vi "FPGA_VI.vi"() -> ()   [LabVIEW 2014]
uses:
  FPGA_Controls/AquisitionState.ctl
  <vilib>/Platform/TimedLoop/XDataNode/timing_clust.ctl
  <vilib>/Platform/TimedLoop/XDataNode/nitl_modes.ctl
  <vilib>/Platform/TimedLoop/XDataNode/wakeup.ctl
  <vilib>/rvi/Emulation/niFpgaSctlEmulationGetInTimedLoop.vi
  <vilib>/rvi/Emulation/niFpgaEmulationReportErrorSimple.vi
  <vilib>/rvi/Emulation/niFpgaGetClockAttributes.vi
  <vilib>/rvi/Emulation/niFpgaCriticalErrorInLSC.vi
  <vilib>/rvi/eio/common/nirviEmuTemplateMethod_errors.vi
  <vilib>/rvi/Emulation/niFpgaProcessEmulError.vi
  <vilib>/rvi/interface/RandomDataEmulation/niFpgaRandomDataHandleErrors.vi
  <vilib>/Platform/TimedLoop/XDataNode/XDataNode.xnode
  <vilib>/eio/EIONode/EIONode.xnode
  <vilib>/rvi/DataTransferAndStorage/Container/XNode/niFpgaContainer.xnode
  <vilib>/rvi/interface/RandomDataEmulation/nirviRandomDataFpgaReadWriteTemplate.vi
  <vilib>/Platform/TimedLoop/XDataNode/XDNodeRunTimeDep.lvlib
panel:
  in  "Trigger":bool
  out "Init Done":bool
  out "Acquisition \nState":T1=enum."Idle (Wait for Trigger)"
  # "ADC"
  # "Status"
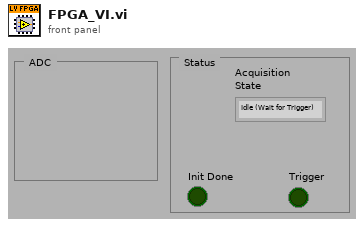
[diagram p1: front panel]
types:
  T1 = typedef "AquisitionState.ctl" = enum16{"Clear DRAM", "Idle (Wait for Trigger)", "Aquire", "Transfer DRAM Block 0", "Transfer DRAM Block 1"}
  T2 = typedef "XDNodeRunTimeDep.lvlib/timing_clust.ctl" = cluster{"Expected End [f-1]":u64, "Actual End [f-1]":u64, "Finished Late? [f-1]":bool, "Expected End [i-1]":u64, "Actual End [i-1]":u64, "Finished Late? [i-1]":bool, "Expected Start [i]":u64, "Actual Start [i]":u64, "Expected Start [f]":u64, "Actual Start [f]":u64, "Source Name":string, "Structure Name":string, "Period":i64, "Deadline":i64, "Offset":i64, "Start":i64, "Priority":i32, "Timeout":i32, "Mode":T3, "Wakeup Reason":T4, "Error":errorcluster, "Source Type":string, "Secondary Source Type":string, "Global End Time":u64, "Global Start Time":u64, "Frame Duration":u64, "Iteration Duration":u64, "Assigned CPU":i32, "I/O Scan Engine Mode":u32}
  T3 = typedef "XDNodeRunTimeDep.lvlib/nitl_modes.ctl" = enum32{"No Change", "Process missed periods, maintain original phase", "Discard missed periods, maintain original phase", "Process missed periods, ignore original phase", "Discard missed periods, ignore original phase"}
  T4 = typedef "XDNodeRunTimeDep.lvlib/wakeup.ctl" = enum32{"Normal", "Aborted", "Asynchronous wakeup", "Timing source error", "Timed loop error", "Timeout"}
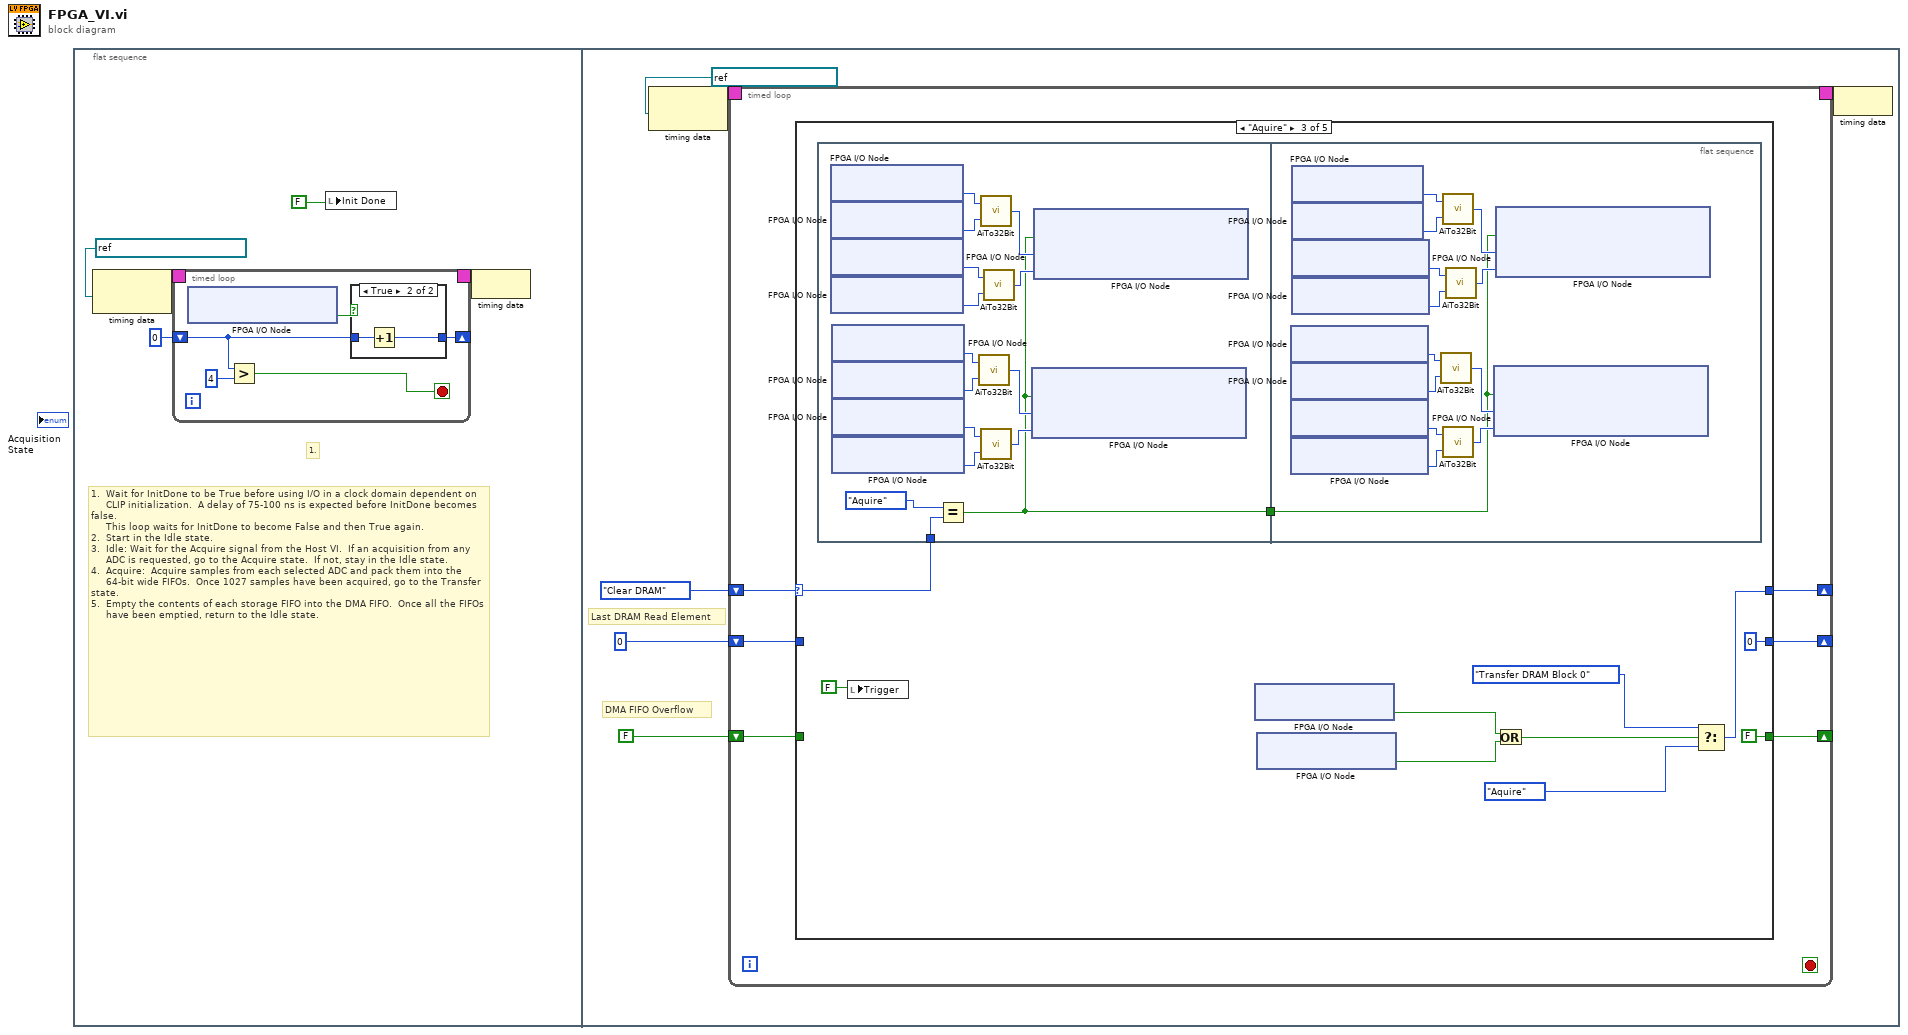
[diagram p0: block diagram]
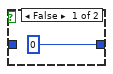
[diagram p2: hidden frame]
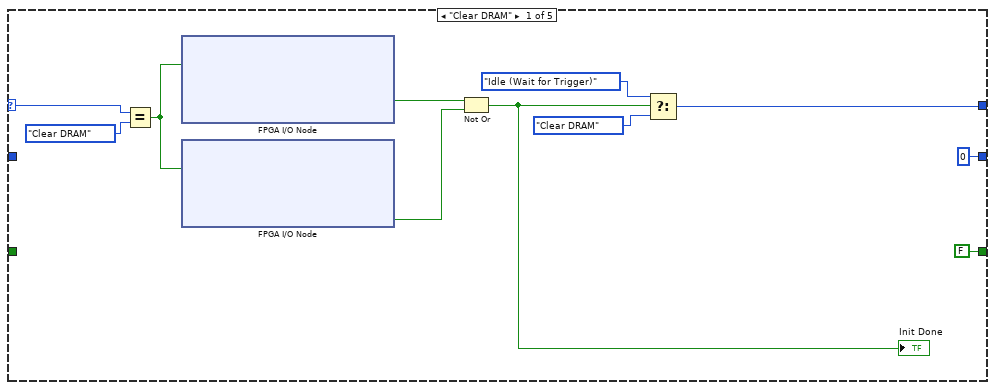
[diagram p3: hidden frame]
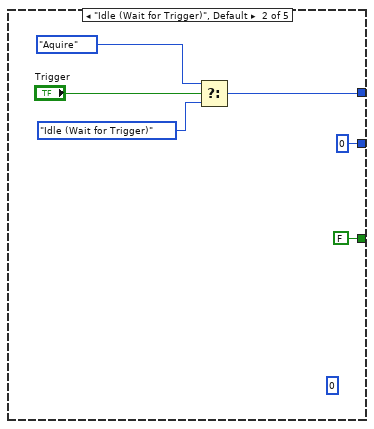
[diagram p4: hidden frame]
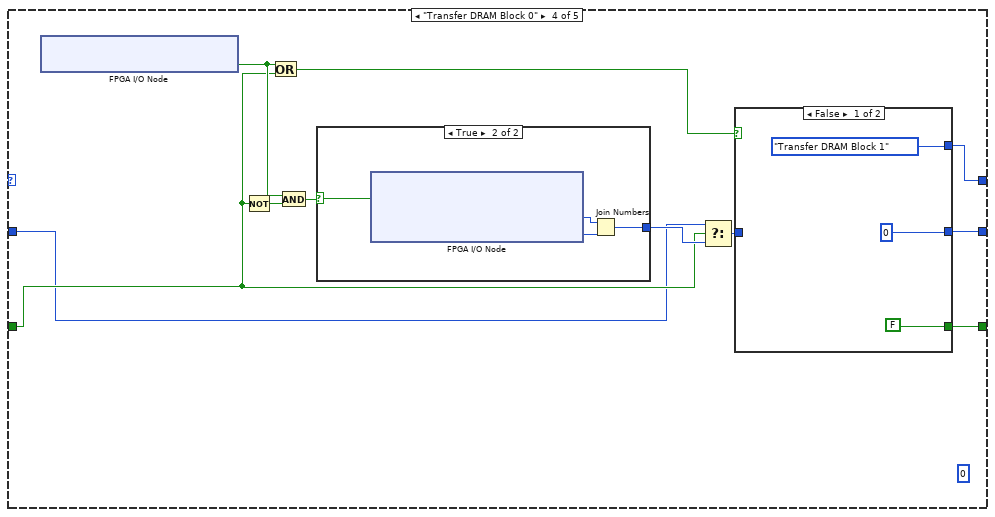
[diagram p5: hidden frame]
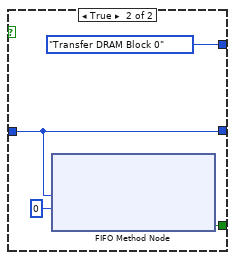
[diagram p6: hidden frame]
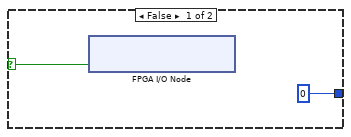
[diagram p7: hidden frame]
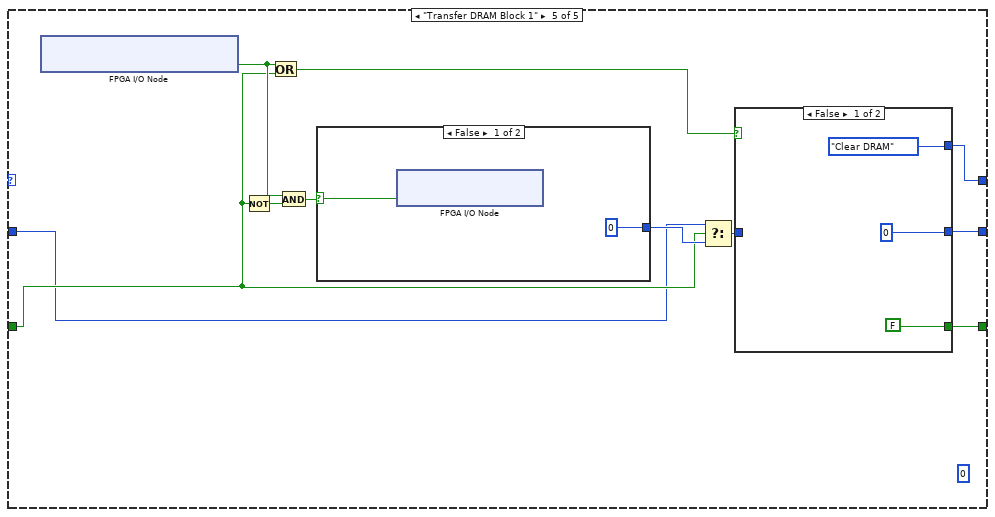
[diagram p8: hidden frame]
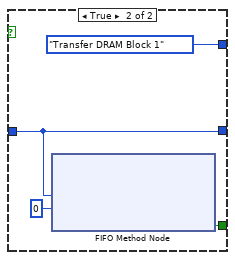
[diagram p9: hidden frame]
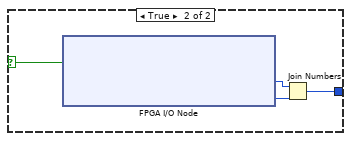
[diagram p10: hidden frame]
diagram:
  n1 = flat-sequence {
    frame #0 {
      # "1.  Wait for InitDone to be True before using I/O in a clock domain dependent on \n     CLIP initialization.  A delay of 75-100 ns is expected before InitDone becomes false.  \n     This loop waits for InitDone to become False and then True again.\n2.  Start in the Idle state. \n3.  Idle: Wait for the Acquire signal from the Host VI.  If an acquisition from any \n     ADC is requested, go to the Acquire state.  If not, stay in the Idle state.\n4.  Acquire:  Acquire samples from each selected ADC and pack them into the  \n     64-bit wide FIFOs.  Once 1027 samples have been acquired, go to the Transfer state.\n5.  Empty the contents of each storage FIFO into the DMA FIFO.  Once all the FIFOs \n     have been emptied, return to the Idle state."
      # "1."
      n2 = node-c288(refnum<k21> "40 MHz Onboard Clock" ("Source Name")) -> (w5:T2)
      n3 = timed-loop {
        shift-right: [w9] -> _
        shift-left: u16 0 -> [w8]
        timing: w5 -> [_]
        timing-out: [_] -> w4
        stop <- w6 stop-if-true
        n4 = xnode "FPGA I/O Node"() -> ("IO Module\\InitDone"=w10:bool)  [unwired: 1 in, 1 out]
        n5 = Greater?(x=w8, y=u16 4) -> (0:w6:bool)
        n6 = case shown="True" w10 {
          tunnel: [u16 0 w13] -> w9
          tunnel: w8 -> [_ w12]
          frame False {
          }
          frame True {
            n7 = Increment(x=w12) -> (x+1=w13:u16)
          }
        }
      }
      n8 = local write "Init Done"(FALSE) -> ()
      n9 = node-c288(w4) -> ()
    }
    frame #1 {
      # "Last DRAM Read Element"
      # "DMA FIFO Overflow"
      n10 = node-c288(refnum<k21> "IO Module Clock 0" ("Source Name")) -> (w25:T2)
      n11 = timed-loop {
        timing: w25 -> [_]
        timing-out: [_] -> w24
        shift-right: [w30] -> _
        shift-left: AquisitionState."Clear DRAM" ("AquistionState") -> [w31]
        shift-right: [w29] -> _
        shift-left: FALSE ("Timed Out?") -> [w27]
        shift-right: [w28] -> _
        shift-left: u64 0 ("Timeout") -> [w26]
        stop <- _ stop-if-true
        n12 = case shown="\"Aquire\"" w31 {
          selector: w31 -> [w42 _ w59 _ _]
          tunnel: [w37 w46 w55 w92 w116] -> w30
          tunnel: [FALSE ("Timed Out?") FALSE ("Timed Out?") FALSE ("Timed Out?") w93 w117] -> w29
          tunnel: [u64 0 ("Timeout") u64 0 ("Timeout") u64 0 ("Timeout") w90 w114] -> w28
          tunnel: w27 -> [_ _ _ w89 w113]
          tunnel: w26 -> [_ _ _ w88 w112]
          frame "Clear DRAM" {
            n13 = Equal?(x=w42, y=AquisitionState."Clear DRAM" ("AquistionState")) -> (x = y?=w40:bool)
            n14 = xnode "FPGA I/O Node"("DRAM Bank 0\\Read"=w40) -> ("DRAM Bank 0\\Data_Available"=w39:bool)  [unwired: 4 in, 6 out]
            n15 = xnode "FPGA I/O Node"("DRAM Bank 1\\Read"=w40) -> ("DRAM Bank 1\\Data_Available"=w38:bool)  [unwired: 4 in, 6 out]
            n16 = Not Or(1:w38, 2:w39) -> (0:w32:bool)
            "Init Done" <- w32
            n17 = Select(t=AquisitionState."Idle (Wait for Trigger)" ("AquistionState"), s=w32, f=AquisitionState."Clear DRAM" ("AquistionState")) -> (s? t:f=w37:T1)
          }
          frame "Idle (Wait for Trigger)", Default {
            (unwired) 0
            n18 = Select(t=AquisitionState."Aquire" ("AquistionState"), s="Trigger", f=AquisitionState."Idle (Wait for Trigger)" ("AquistionState")) -> (s? t:f=w46:T1)
          }
          frame "Aquire" {
            n19 = flat-sequence {
              tunnel: w59 -> [w62]
              tunnel: [w60] -> w58
              tunnel: w58 -> [w75]
              frame #0 {
                n20 = xnode "FPGA I/O Node"() -> ("IO Module\\AI A0"=w74:i16)  [unwired: 1 in, 1 out]
                n21 = xnode "FPGA I/O Node"() -> ("IO Module\\AI A1"=w73:i16)  [unwired: 1 in, 1 out]
                n22 = xnode "FPGA I/O Node"() -> ("IO Module\\AI A2"=w72:i16)  [unwired: 1 in, 1 out]
                n23 = xnode "FPGA I/O Node"() -> ("IO Module\\AI A3"=w71:i16)  [unwired: 1 in, 1 out]
                n24 = xnode "FPGA I/O Node"() -> ("IO Module\\AI A4"=w67:i16)  [unwired: 1 in, 1 out]
                n25 = xnode "FPGA I/O Node"() -> ("IO Module\\AI A5"=w66:i16)  [unwired: 1 in, 1 out]
                n26 = xnode "FPGA I/O Node"() -> ("IO Module\\AI A6"=w65:i16)  [unwired: 1 in, 1 out]
                n27 = xnode "FPGA I/O Node"() -> ("IO Module\\AI A7"=w64:i16)  [unwired: 1 in, 1 out]
                n28 = Equal?(x=AquisitionState."Aquire" ("AquistionState"), y=w62) -> (x = y?=w60:bool)
                n29 = call "AiTo32Bit.vi"("AI 0"=w66, "AI 1"=w67) -> ("AI 32bit"=w63:u32)
                n30 = call "AiTo32Bit.vi"("AI 0"=w73, "AI 1"=w74) -> ("AI 32bit"=w69:u32)
                n31 = call "AiTo32Bit.vi"("AI 0"=w64, "AI 1"=w65) -> ("AI 32bit"=w68:u32)
                n32 = call "AiTo32Bit.vi"("AI 0"=w71, "AI 1"=w72) -> ("AI 32bit"=w70:u32)
                n33 = xnode "FPGA I/O Node"("DRAM Bank 1\\Write"=w60, "DRAM Bank 1\\Write_Data_Upper"=w63, "DRAM Bank 1\\Write_Data_Lower"=w68) -> ()  [unwired: 3 in, 3 out]
                n34 = xnode "FPGA I/O Node"("DRAM Bank 0\\Write"=w60, "DRAM Bank 0\\Write_Data_Upper"=w69, "DRAM Bank 0\\Write_Data_Lower"=w70) -> ()  [unwired: 3 in, 3 out]
              }
              frame #1 {
                n35 = xnode "FPGA I/O Node"() -> ("IO Module\\AI B12"=w79:i16)  [unwired: 1 in, 1 out]
                n36 = xnode "FPGA I/O Node"() -> ("IO Module\\AI B13"=w78:i16)  [unwired: 1 in, 1 out]
                n37 = xnode "FPGA I/O Node"() -> ("IO Module\\AI B14"=w77:i16)  [unwired: 1 in, 1 out]
                n38 = xnode "FPGA I/O Node"() -> ("IO Module\\AI B15"=w76:i16)  [unwired: 1 in, 1 out]
                n39 = xnode "FPGA I/O Node"() -> ("IO Module\\AI B8"=w83:i16)  [unwired: 1 in, 1 out]
                n40 = xnode "FPGA I/O Node"() -> ("IO Module\\AI B9"=w82:i16)  [unwired: 1 in, 1 out]
                n41 = xnode "FPGA I/O Node"() -> ("IO Module\\AI B10"=w81:i16)  [unwired: 1 in, 1 out]
                n42 = xnode "FPGA I/O Node"() -> ("IO Module\\AI B11"=w80:i16)  [unwired: 1 in, 1 out]
                n43 = call "AiTo32Bit.vi"("AI 0"=w78, "AI 1"=w79) -> ("AI 32bit"=w84:u32)
                n44 = call "AiTo32Bit.vi"("AI 0"=w82, "AI 1"=w83) -> ("AI 32bit"=w86:u32)
                n45 = call "AiTo32Bit.vi"("AI 0"=w76, "AI 1"=w77) -> ("AI 32bit"=w85:u32)
                n46 = call "AiTo32Bit.vi"("AI 0"=w80, "AI 1"=w81) -> ("AI 32bit"=w87:u32)
                n47 = xnode "FPGA I/O Node"("DRAM Bank 1\\Write"=w75, "DRAM Bank 1\\Write_Data_Upper"=w84, "DRAM Bank 1\\Write_Data_Lower"=w85) -> ()  [unwired: 3 in, 3 out]
                n48 = xnode "FPGA I/O Node"("DRAM Bank 0\\Write"=w75, "DRAM Bank 0\\Write_Data_Upper"=w86, "DRAM Bank 0\\Write_Data_Lower"=w87) -> ()  [unwired: 3 in, 3 out]
              }
            }
            n49 = local write "Trigger"(FALSE) -> ()
            n50 = xnode "FPGA I/O Node"() -> ("DRAM Bank 0\\Full"=w51:bool)  [unwired: 1 in, 1 out]
            n51 = xnode "FPGA I/O Node"() -> ("DRAM Bank 1\\Full"=w50:bool)  [unwired: 1 in, 1 out]
            n52 = Or(x=w51, y=w50) -> (x .or. y?=w52:bool)
            n53 = Select(t=AquisitionState."Transfer DRAM Block 0" ("AquistionState"), s=w52, f=AquisitionState."Aquire" ("AquistionState")) -> (s? t:f=w55:T1)
          }
          frame "Transfer DRAM Block 0" {
            (unwired) 0
            n54 = xnode "FPGA I/O Node"() -> ("DRAM Bank 0\\Data_Available"=w96:bool)  [unwired: 1 in, 1 out]
            n55 = Not(x=w89) -> (.not. x?=w97:bool)
            n56 = Or(x=w96, y=w89) -> (x .or. y?=w91:bool)
            n57 = And(x=w96, y=w97) -> (x .and. y?=w98:bool)
            n58 = case shown="True" w98 {
              selector: w98 -> [w106 w109]
              tunnel: [u64 0 ("Timeout") w108] -> w95
              frame False {
                n59 = xnode "FPGA I/O Node"("DRAM Bank 0\\Read"=w106) -> ()  [unwired: 1 in, 1 out]
              }
              frame True {
                n60 = xnode "FPGA I/O Node"("DRAM Bank 0\\Read"=w109) -> ("DRAM Bank 0\\Read_Data_Upper"=w110:u32, "DRAM Bank 0\\Read_Data_Lower"=w111:u32)  [unwired: 3 in, 3 out]
                n61 = Join Numbers(hi=w110, lo=w111) -> ((hi.lo)=w108:u64)
              }
            }
            n62 = Select(t=w88, s=w89, f=w95) -> (s? t:f=w94:u64)
            n63 = case shown="False" w91 {
              tunnel: [FALSE ("Timed Out?") w105] -> w93
              tunnel: [u64 0 ("Timeout") w102] -> w90
              tunnel: [AquisitionState."Transfer DRAM Block 1" ("Acquisition State 2") AquisitionState."Transfer DRAM Block 0" ("Acquisition State 2")] -> w92
              tunnel: w94 -> [_ w102]
              frame False {
              }
              frame True {
                n64 = xnode ("FIFO Method Node")("Element"=w102, "Timeout"=0) -> ("Timed Out?"=w105:bool)  [unwired: 1 in, 1 out]
              }
            }
          }
          frame "Transfer DRAM Block 1" {
            (unwired) 0
            n65 = xnode "FPGA I/O Node"() -> ("DRAM Bank 1\\Data_Available"=w120:bool)  [unwired: 1 in, 1 out]
            n66 = Not(x=w113) -> (.not. x?=w121:bool)
            n67 = Or(x=w120, y=w113) -> (x .or. y?=w115:bool)
            n68 = And(x=w120, y=w121) -> (x .and. y?=w122:bool)
            n69 = case shown="False" w122 {
              selector: w122 -> [w130 w133]
              tunnel: [u64 0 ("Timeout") w132] -> w119
              frame False {
                n70 = xnode "FPGA I/O Node"("DRAM Bank 1\\Read"=w130) -> ()  [unwired: 1 in, 1 out]
              }
              frame True {
                n71 = xnode "FPGA I/O Node"("DRAM Bank 1\\Read"=w133) -> ("DRAM Bank 1\\Read_Data_Upper"=w134:u32, "DRAM Bank 1\\Read_Data_Lower"=w135:u32)  [unwired: 3 in, 3 out]
                n72 = Join Numbers(hi=w134, lo=w135) -> ((hi.lo)=w132:u64)
              }
            }
            n73 = Select(t=w112, s=w113, f=w119) -> (s? t:f=w118:u64)
            n74 = case shown="False" w115 {
              tunnel: [FALSE ("Timed Out?") w129] -> w117
              tunnel: [u64 0 ("Timeout") w126] -> w114
              tunnel: [AquisitionState."Clear DRAM" ("Acquisition State 2") AquisitionState."Transfer DRAM Block 1" ("Acquisition State 2")] -> w116
              tunnel: w118 -> [_ w126]
              frame False {
              }
              frame True {
                n75 = xnode ("FIFO Method Node")("Element"=w126, "Timeout"=0) -> ("Timed Out?"=w129:bool)  [unwired: 1 in, 1 out]
              }
            }
          }
        }
      }
      n76 = node-c288(w24) -> ()
    }
  }
